vi "мультиплексор(2 4-разрядных операнда).vi"(1 "c":bool, 2 "B":T2, 3 "A":T3) -> (0 "R":T1)   [LabVIEW 2013]
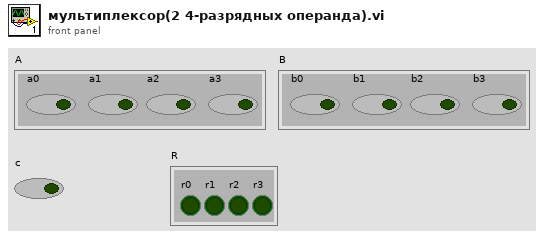
[diagram p1: front panel]
types:
  T1 = cluster{"r0":bool, "r1":bool, "r2":bool, "r3":bool}
  T2 = cluster{"b0":bool, "b1":bool, "b2":bool, "b3":bool}
  T3 = cluster{"a0":bool, "a1":bool, "a2":bool, "a3":bool}
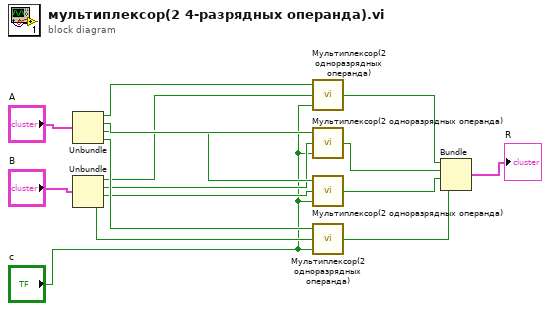
[diagram p0: block diagram]
diagram:
  n1 = Unbundle("A") -> ("a0"=w15:bool, "a1"=w14:bool, "a2"=w13:bool, "a3"=w12:bool)
  n2 = Unbundle("B") -> ("b0"=w10:bool, "b1"=w9:bool, "b2"=w8:bool, "b3"=w7:bool)
  n3 = call "Мультиплексор(2 одноразрядных операнда).vi"("c"="c", "y"=w10, "x"=w15) -> ("r"=w4:bool)
  n4 = call "Мультиплексор(2 одноразрядных операнда).vi"("c"="c", "y"=w9, "x"=w14) -> ("r"=w3:bool)
  n5 = call "Мультиплексор(2 одноразрядных операнда).vi"("c"="c", "y"=w8, "x"=w13) -> ("r"=w2:bool)
  n6 = call "Мультиплексор(2 одноразрядных операнда).vi"("c"="c", "y"=w7, "x"=w12) -> ("r"=w1:bool)
  n7 = Bundle("r"=w4, "r"=w3, "r"=w2, "r"=w1) -> (→"R":cluster{"r":bool, "r":bool, "r":bool, "r":bool})  [unwired: 1 in]
